vi "templates TEMPLATE data keys.vi"(4 "sxUsername":string, 6 "POST Parameters":T1, 7 "HTM Keys":T1, 8 "error in (no error)":errorcluster, 9 "Template Parameters":T1, 10 "Template Record":T3, 11 "Connection Refnum":T2) -> (0 "error out":errorcluster, 2 "Template Keys":T1, 3 "Connection Refnum":T2, 5 "HTM Keys":T1)   [LabVIEW 2011]
uses:
  ITK EXT/utils/keyedarr.llb/Keyed Array.ctl
  server/database/Templates/Template Record.ctl
  Summitek EXT/ODBC/SQL Controls/Connection Refnum.ctl
  ITK EXT/utils/strutil.llb/Case Matching.ctl
  Summitek EXT/OpenG EXT/file/file.llb/Strip Path Extension - String__ogtk.vi
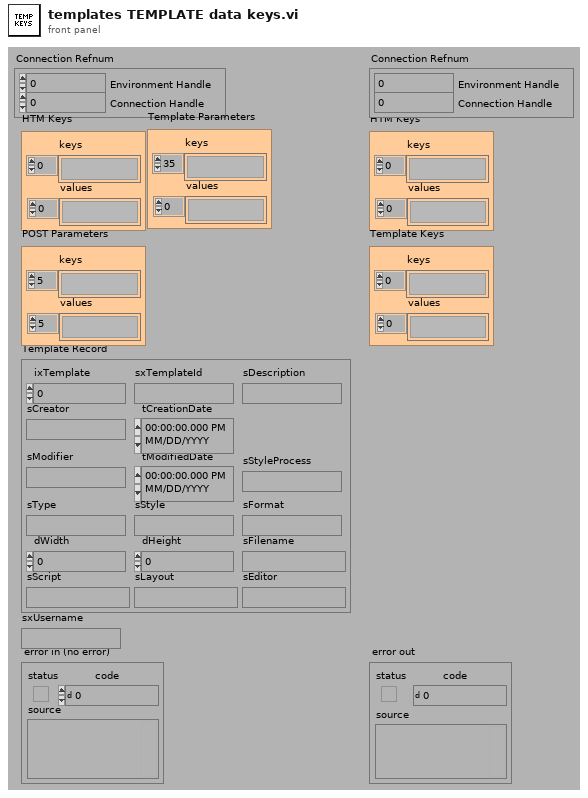
[diagram p1: front panel]
types:
  T1 = typedef "Keyed Array.ctl" = cluster{"keys":string[], "values":string[]}
  T2 = typedef "Connection Refnum.ctl" = cluster{"Environment Handle":i32, "Connection Handle":i32}
  T3 = typedef "Template Record.ctl" = cluster{"ixTemplate":i32, "sxTemplateId":string, "sDescription":string, "sCreator":string, "tCreationDate":timestamp, "sModifier":string, "tModifiedDate":timestamp, "sType":string, "sStyle":string, "sFormat":string, "dWidth":dbl, "dHeight":dbl, "sFilename":string, "sScript":string, "sLayout":string, "sEditor":string, "sStyleProcess":string}
  T4 = typedef "Case Matching.ctl" = enum16{"a != A", "a == A", "system"}
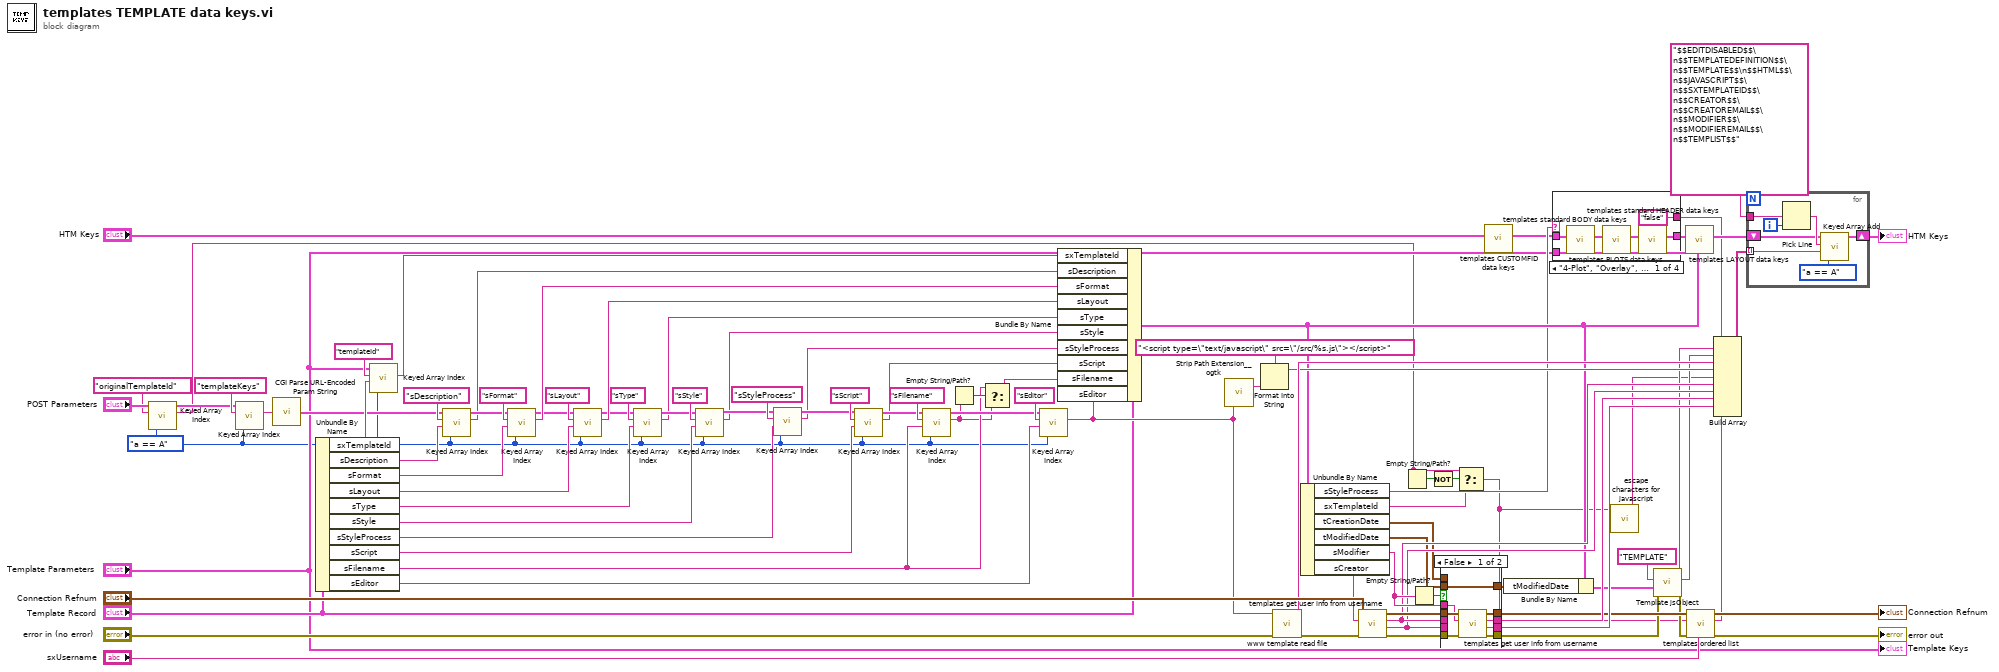
[diagram p0: block diagram]
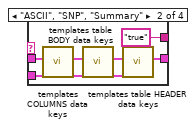
[diagram p2: hidden frame]
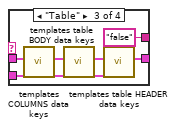
[diagram p3: hidden frame]
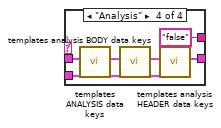
[diagram p4: hidden frame]
diagram:
  w14 = Case_Matching."a == A" ("case matching (sensitive)")
  n1 = call "Keyed Array Index.vi"("case matching (sensitive)"=w14, "key"="originalTemplateId", "array in"="POST Parameters") -> ("value"=w6:string, "duplicate array"=w13:T1)  [unwired: 1 in, 2 out]
  n2 = call "Keyed Array Index.vi"("case matching (sensitive)"=w14, "key"="templateKeys", "array in"=w13) -> ("value"=w72:string)  [unwired: 1 in, 3 out]
  n3 = call "CGI Parse URL-Encoded Param String.vi"("url-encoded param string"=w72) -> ("params"=w23:T1)
  n4 = Unbundle By Name("Template Record") -> ("sxTemplateId"=w25:string, "sDescription"=w34:string, "sFormat"=w35:string, "sLayout"=w36:string, "sType"=w67:string, "sStyle"=w66:string, "sStyleProcess"=w22:string, "sScript"=w65:string, "sFilename"=w29:string, "sEditor"=w54:string)
  n5 = call "Keyed Array Index.vi"("case matching (sensitive)"=w14, "default value"=w25, "key"="templateId", "array in"="Template Parameters") -> ("value"=w26:string)  [unwired: 3 out]
  n6 = call "Keyed Array Index.vi"("case matching (sensitive)"=w14, "default value"=w34, "key"="sDescription", "array in"=w23) -> ("value"=w37:string, "duplicate array"=w40:T1)  [unwired: 2 out]
  n7 = call "Keyed Array Index.vi"("case matching (sensitive)"=w14, "default value"=w35, "key"="sFormat", "array in"=w40) -> ("value"=w41:string, "duplicate array"=w39:T1)  [unwired: 2 out]
  n8 = call "Keyed Array Index.vi"("case matching (sensitive)"=w14, "default value"=w36, "key"="sLayout", "array in"=w39) -> ("value"=w42:string, "duplicate array"=w38:T1)  [unwired: 2 out]
  n9 = call "Keyed Array Index.vi"("case matching (sensitive)"=w14, "default value"=w67, "key"="sType", "array in"=w38) -> ("value"=w5:string, "duplicate array"=w68:T1)  [unwired: 2 out]
  n10 = call "Keyed Array Index.vi"("case matching (sensitive)"=w14, "default value"=w66, "key"="sStyle", "array in"=w68) -> ("value"=w4:string, "duplicate array"=w20:T1)  [unwired: 2 out]
  n11 = call "Keyed Array Index.vi"("case matching (sensitive)"=w14, "default value"=w22, "key"="sStyleProcess", "array in"=w20) -> ("value"=w3:string, "duplicate array"=w19:T1)  [unwired: 2 out]
  n12 = call "Keyed Array Index.vi"("case matching (sensitive)"=w14, "default value"=w65, "key"="sScript", "array in"=w19) -> ("value"=w1:string, "duplicate array"=w18:T1)  [unwired: 2 out]
  n13 = call "Keyed Array Index.vi"("case matching (sensitive)"=w14, "default value"=w29, "key"="sFilename", "array in"=w18) -> ("value"=w28:string, "duplicate array"=w56:T1)  [unwired: 2 out]
  n14 = Empty String/Path?(string/path=w28) -> (empty?=w30:bool)
  n15 = Select(t=w29, s=w30, f=w28) -> (s? t:f=w2:string)
  n16 = call "Keyed Array Index.vi"("case matching (sensitive)"=w14, "default value"=w54, "key"="sEditor", "array in"=w56) -> ("value"=w55:string)  [unwired: 3 out]
  n17 = Bundle By Name(cluster="Template Record", "sxTemplateId"=w26, "sDescription"=w37, "sFormat"=w41, "sLayout"=w42, "sType"=w5, "sStyle"=w4, "sStyleProcess"=w3, "sScript"=w1, "sFilename"=w2, "sEditor"=w55) -> (w48:T3)
  n18 = call-poly "Strip Path Extension__ogtk.vi"("path"=w55) -> ("root"=w77:string)  [unwired: 1 out]
  n19 = Format Into String(format string="<script type=\"text/javascript\" src=\"/src/%s.js\"></script>", w77) -> (resulting string=w74:string)  [unwired: 2 in, 1 out]
  n20 = call "www template read file.vi"("error in (no error)"="error in (no error)", "Template File (\"\")"=w55) -> ("error out"=w79:errorcluster, "Page HTML"=w81:string)  [unwired: 2 in, 6 out]
  n21 = Unbundle By Name(w48) -> ("sStyleProcess"=w33:string, "sxTemplateId"=w7:string, "tCreationDate"=w76:timestamp, "tModifiedDate"=w80:timestamp, "sModifier"=w90:string, "sCreator"=w91:string)
  n22 = call "templates get user info from username.vi"("error in (no error)"=w79, "Username (\"\")"=w91, "Connection Refnum"="Connection Refnum") -> ("error out"=w94:errorcluster, "Email"=w87:string, "First Last"=w88:string, "Connection Refnum"=w95:T2)  [unwired: 5 out]
  n23 = Empty String/Path?(string/path=w6) -> (empty?=w10:bool)
  n24 = Empty String/Path?(string/path=w90) -> (empty?=w93:bool)
  n25 = Not(x=w10) -> (.not. x?=w8:bool)
  n26 = case shown="False" w93 {
    tunnel: w95 -> [w103 w107]
    tunnel: w94 -> [w102 w106]
    tunnel: w90 -> [w101 _]
    tunnel: w88 -> [_ w105]
    tunnel: w87 -> [_ w104]
    tunnel: w80 -> [w98 _]
    tunnel: [w98 w108] -> w47
    tunnel: [w100 w107] -> w61
    tunnel: [w99 w106] -> w53
    tunnel: w76 -> [_ w108]
    tunnel: [w97 w105] -> w86
    tunnel: [w96 w104] -> w85
    frame False {
      n27 = call "templates get user info from username.vi"("error in (no error)"=w102, "Username (\"\")"=w101, "Connection Refnum"=w103) -> ("error out"=w99:errorcluster, "Email"=w96:string, "First Last"=w97:string, "Connection Refnum"=w100:T2)  [unwired: 5 out]
    }
    frame True {
    }
  }
  n28 = Select(t=w6, s=w8, f=w7) -> (s? t:f=w9:string)
  n29 = call "templates CUSTOMFID data keys.vi"("Template Keys"="Template Parameters", "HTM Keys"="HTM Keys") -> ("HTM Keys"=w17:T1)  [unwired: 9 out]
  n30 = Bundle By Name(cluster=w48, "tModifiedDate"=w47) -> (w46:T3)
  n31 = case shown="\"4-Plot\", \"Overlay\", Default" w33 {
    tunnel: w17 -> [w114 w120 w126 w132]
    tunnel: [w111 w116 w122 w129] -> w75
    tunnel: "Template Parameters" -> [w110 w118 w124 w128]
    tunnel: ["false" ("key") "true" ("key") "false" ("key") "false" ("key")] -> w64
    frame "4-Plot", "Overlay", Default {
      n32 = call "templates PLOTS data keys.vi"("Template Keys"=w110, "HTM Keys"=w114) -> ("HTM Keys"=w113:T1)  [unwired: 9 out]
      n33 = call "templates standard BODY data keys.vi"("Template Keys"=w110, "HTM Keys"=w113) -> ("HTM Keys"=w112:T1)  [unwired: 9 out]
      n34 = call "templates standard HEADER data keys.vi"("Template Keys"=w110, "HTM Keys"=w112) -> ("HTM Keys"=w111:T1)  [unwired: 9 out]
    }
    frame "ASCII", "SNP", "Summary" {
      n35 = call "templates COLUMNS data keys.vi"("Template Keys"=w118, "HTM Keys"=w120) -> ("HTM Keys"=w119:T1)  [unwired: 9 out]
      n36 = call "templates table BODY data keys.vi"("Template Keys"=w118, "HTM Keys"=w119) -> ("HTM Keys"=w117:T1)  [unwired: 9 out]
      n37 = call "templates table HEADER data keys.vi"("Template Keys"=w118, "HTM Keys"=w117) -> ("HTM Keys"=w116:T1)  [unwired: 9 out]
    }
    frame "Table" {
      n38 = call "templates COLUMNS data keys.vi"("Template Keys"=w124, "HTM Keys"=w126) -> ("HTM Keys"=w125:T1)  [unwired: 9 out]
      n39 = call "templates table BODY data keys.vi"("Template Keys"=w124, "HTM Keys"=w125) -> ("HTM Keys"=w123:T1)  [unwired: 9 out]
      n40 = call "templates table HEADER data keys.vi"("Template Keys"=w124, "HTM Keys"=w123) -> ("HTM Keys"=w122:T1)  [unwired: 9 out]
    }
    frame "Analysis" {
      n41 = call "templates ANALYSIS data keys.vi"("Template Keys"=w128, "HTM Keys"=w132) -> ("HTM Keys"=w131:T1)  [unwired: 9 out]
      n42 = call "templates analysis BODY data keys.vi"("Template Keys"=w128, "HTM Keys"=w131) -> ("HTM Keys"=w130:T1)  [unwired: 1 in, 8 out]
      n43 = call "templates analysis HEADER data keys.vi"("Template Keys"=w128, "HTM Keys"=w130) -> ("HTM Keys"=w129:T1)  [unwired: 9 out]
    }
  }
  n44 = call "escape characters for javascript.vi"("String (\"\")"=w9) -> ("escaped String"=w24:string)  [unwired: 4 out]
  n45 = call "Template jsObject.vi"("error in (no error)"=w53, "Template Record (empty)"=w46, "Template jsObject Name (\"\")"="TEMPLATE") -> ("error out"=w52:errorcluster, "Template jsObject"=w50:string, "Template jsObject Definition"=w51:string)  [unwired: 1 in, 5 out]
  n46 = call "templates LAYOUT data keys.vi"("Template Record"=w48, "Template Keys"="Template Parameters", "HTM Keys"=w75) -> ("HTM Keys"=w82:T1)  [unwired: 8 out]
  n47 = call "templates ordered list.vi"("sxUsername"="sxUsername", "error in (no error)"=w52, "sxTemplateId (\"\")"=w9, "Connection Refnum"=w61) -> ("error out"=→"error out":errorcluster, "Templates List"=w60:string, "Connection Refnum"=→"Connection Refnum":T2)  [unwired: 5 out]
  n48 = Build Array(w64, w51, w50, w81, w74, w24, w88, w87, w86, w85, w60) -> (w84:string[])
  n49 = for {
    shift-right: [w135] -> w83
    shift-left: w82 -> [w136]
    tunnel: "$$EDITDISABLED$$\n$$TEMPLATEDEFINITION$$\n$$TEMPLATE$$\n$$HTML$$\n$$JAVASCRIPT$$\n$$SXTEMPLATEID$$\n$$CREATOR$$\n$$CREATOREMAIL$$\n$$MODIFIER$$\n$$MODIFIEREMAIL$$\n$$TEMPLIST$$" ("key") -> [w134]
    tunnel: w84 -> [w133] mode=indexing
    i -> [w138]
    n50 = Pick Line(multi-line string=w134, line index=w138) -> (output string=w137:string)  [unwired: 1 out]
    n51 = call "Keyed Array Add.vi"("case matching (sensitive)"=Case_Matching."a == A", "value"=w133, "key"=w137, "array in"=w136) -> ("array out"=w135:T1)  [unwired: 3 out]
  }
  "HTM Keys" <- w83
  "Template Keys" <- "Template Parameters"
